vi "Global Strings.vi"() -> ()   [LabVIEW 2020, in "Sequencer with Output Values.lvlib" / "Sequencer with Output Values.lvclass"]
uses:
  Sequencer with Output Values.lvclass
panel:
  in  "Delimeter":string=";"
  out "Test Running":bool
  in  "Digital Channel Name":string="Digital Channel %d"
  in  "Analog Channel Name":string="Analog Channel %d"
  in  "Default Mode Value":string="Wait for end of step"
  in  "Mode Enum Values":string[](array[string])=["Wait for end of step", "Repeat channel values"]
  in  "Step Delay Between Values":string="Step %d - Delay between values (use 0 to space evenly)"
  in  "Step Digital Values":string="Step %d - Digital channel %d values (use ; between values)"
  in  "Step Analog Values":string="Step %d - Analog channel %d values (use ; between values)"
  in  "Step Mode":string="Step %d - Update channel mode"
  in  "Number of Digital Channels":string="Number of digital channels"
  in  "Number of Analog Channels":string="Number of analog channels"
  in  "Delay Before Starting Sequence":string="Delay before starting sequence (seconds)"
  in  "Step Duration":string="Step %d - Duration (seconds)"
  in  "Number of Sequence Steps":string="Number of sequence steps"
  in  "Only Execute When Test Running":string="Only execute sequence when test running"
  # "Sequence settings"
  # "Step Settings"
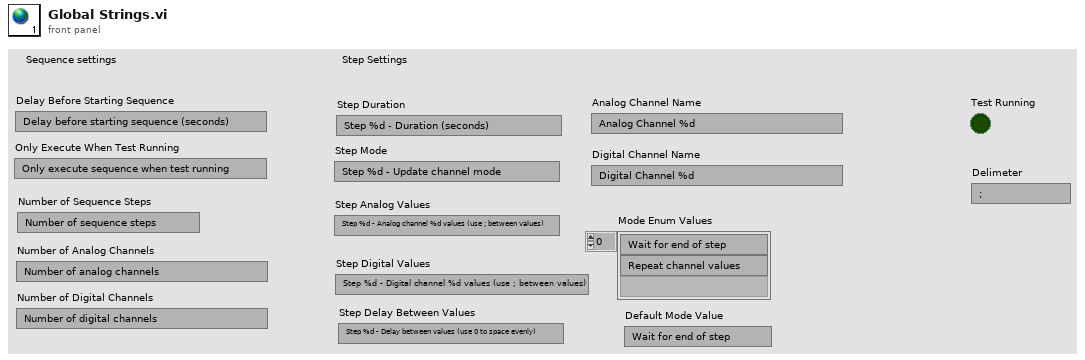
[diagram p1: front panel]
diagram:
